vi "zad2Zmienna.vi"() -> ()   [LabVIEW 2017]
panel:
  out "czyStop 2":bool
  out "czyStop 1":bool
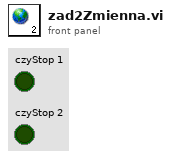
[diagram p1: front panel]
diagram:
